vi "data_lv2gbl.vi"(0 "Data":u64, 5 "Operations":T1=enum."Get_array", 7 "Stop_in":bool=TRUE, 11 "error in":errorcluster) -> (4 "Data out":u64[](array[numeric]), 6 "Last_val":u64, 8 "Stop_out":bool=TRUE, 15 "error out":errorcluster)   [LabVIEW 2023, in "task-1.lvlib"]
doc: "A LV2GBl to store the data values."
uses:
  controls/Operations.ctl
  task-1.lvlib
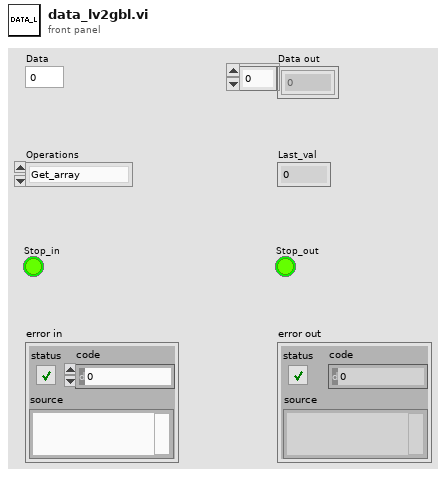
[diagram p1: front panel]
types:
  T1 = typedef "task-1.lvlib/Operations.ctl" = enum16{"Set_Stop", "Get_array", "Get_last_val", "Add_val", "Initialize"}
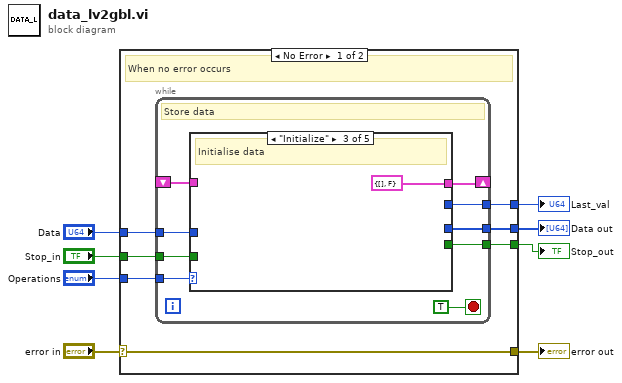
[diagram p0: block diagram]
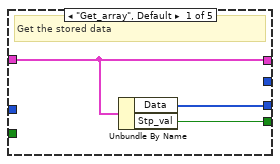
[diagram p2: hidden frame]
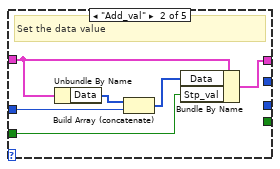
[diagram p3: hidden frame]
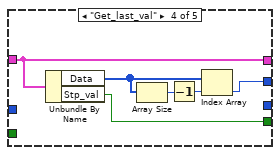
[diagram p4: hidden frame]
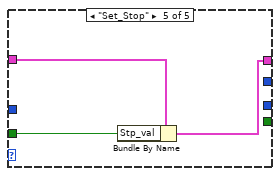
[diagram p5: hidden frame]
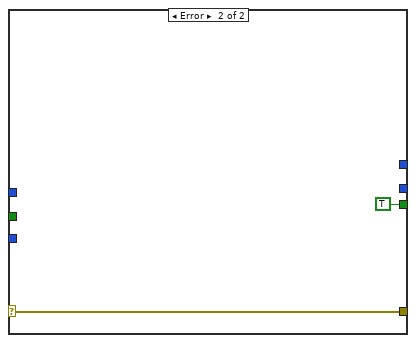
[diagram p6: hidden frame]
diagram:
  n1 = case shown="No Error" "error in" {
    selector: "error in" -> [w15 w45]
    tunnel: [w15 w45] -> w7
    tunnel: "Data" -> [w13 _]
    tunnel: "Operations" -> [w14 _]
    tunnel: [w12 _] -> w4
    tunnel: [w11 _] -> w3
    tunnel: [w10 TRUE ("Stp_val")] -> w2
    tunnel: "Stop_in" -> [w9 _]
    frame No Error {
      # "When no error occurs"
      n2 = while {
        shift-right: [w19] -> _
        shift-left: _ -> [w23]
        tunnel: w14 -> [w24]
        tunnel: w13 -> [w21]
        tunnel: [w20] -> w12
        tunnel: [w18] -> w11
        tunnel: [w17] -> w10
        tunnel: w9 -> [w16]
        stop <- TRUE stop-if-true
        # "Store data"
        n3 = case shown="\"Initialize\"" w24 {
          tunnel: w23 -> [w27 w31 _ w39 w43]
          tunnel: w21 -> [_ w33 _ _ _]
          tunnel: [_ _ _ w40 _] -> w20
          tunnel: [w27 w29 cluster{"Data":u64[], "Stp_val":bool} {"Data"=[], "Stp_val"=FALSE} w39 w41] -> w19
          tunnel: [w26 _ _ _ _] -> w18
          tunnel: [w25 _ _ w38 _] -> w17
          tunnel: w16 -> [_ w28 _ _ w42]
          frame "Get_array", Default {
            # "Get the stored data"
            n4 = Unbundle By Name(w27) -> ("Data"=w26:u64[], "Stp_val"=w25:bool)
          }
          frame "Add_val" {
            # "Set the data value"
            n5 = Unbundle By Name(w31) -> ("Data"=w32:u64[])
            n6 = Build Array (concatenate)(w32, w33) -> (w30:u64[])
            n7 = Bundle By Name(cluster=w31, "Data"=w30, "Stp_val"=w28) -> (w29:cluster{"Data":u64[], "Stp_val":bool})
          }
          frame "Initialize" {
            # "Initialise data"
          }
          frame "Get_last_val" {
            n8 = Unbundle By Name(w39) -> ("Data"=w37:u64[], "Stp_val"=w38:bool)
            n9 = Array Size(array=w37) -> (size(s)=w36:i32)
            n10 = Decrement(x=w36) -> (x-1=w35:i32)
            n11 = Index Array(array=w37, index=w35) -> (element=w40:u64)
          }
          frame "Set_Stop" {
            n12 = Bundle By Name(cluster=w43, "Stp_val"=w42) -> (w41:cluster{"Data":u64[], "Stp_val":bool})
          }
        }
      }
    }
    frame Error {
    }
  }
  "error out" <- w7
  "Data out" <- w3
  "Last_val" <- w4
  "Stop_out" <- w2
